vi "Three Pins Test.vi"() -> ()   [LabVIEW 2012]
panel:
  in  "VI路径":path
  out "Data Table":string[][](table)
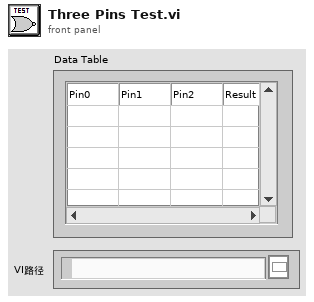
[diagram p1: front panel]
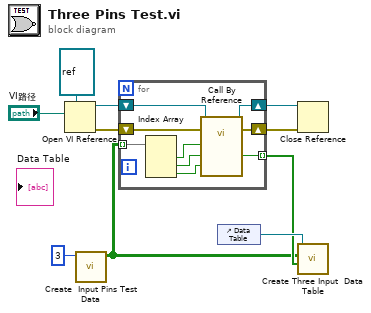
[diagram p0: block diagram]
diagram:
  n1 = Open VI Reference(type specifier VI Refnum (for type only)=refnum<vi> refnum ("类型说明符VI引用句柄（仅用于类型）"), vi path="VI路径") -> (vi reference=w7:refnum<vi>, error out=w6:errorcluster)  [unwired: 4 in]
  n2 = call "Create  Input Pins Test Data.vi"("Pins Num"=3) -> ("Data"=w1:bool[][])  [unwired: 9 in, 1 out]
  n3 = for {
    tunnel: w1 -> [w19] mode=indexing
    tunnel: [w16] -> w9 mode=indexing
    shift-right: [w15] -> w5
    shift-left: w6 -> [w14]
    shift-right: [w13] -> w4
    shift-left: w7 -> [w12]
    n4 = Index Array(array=w19) -> (element #1=w18:bool, element #2=w17:bool, element #3=w11:bool)  [unwired: 3 in]
    n5 = call-by-ref "?"(reference=w12, error in=w14, "Pin2"=w11, "Pin1"=w17, "Pin0"=w18) -> (reference out=w13:refnum<vi>, error out=w15:errorcluster, "Output"=w16:bool)
  }
  n6 = control-ref of="Data Table"() -> (w10:refnum<vi>)
  n7 = Close Reference(reference=w4, error in (no error)=w5) -> ()  [unwired: 1 out]
  n8 = call "Create Three Input  Data Table.vi"("Result"=w9, "Data"=w1, "Data Table Ref In"=w10) -> ()  [unwired: 7 in, 2 out]
